vi "02reg_path_file.vi"(1 "Nombre":string, 2 "Nº equipo":i32, 3 "Exe path":string) -> (0 "file path nvo":path=path "C:/Documents and Settings/All Users/Documentos/LabVIEW Data/Soft Telemedicion/Beta 2.2/Equipo1/09-06-18.xls")   [LabVIEW 2010]
uses:
  <vilib>/Utility/file.llb/Read From Spreadsheet File (DBL).vi
panel:
  out "error out":errorcluster
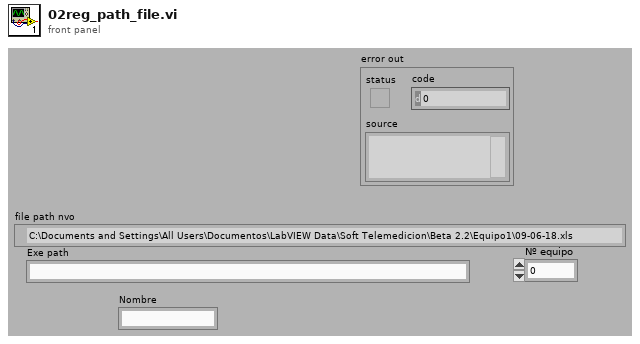
[diagram p1: front panel]
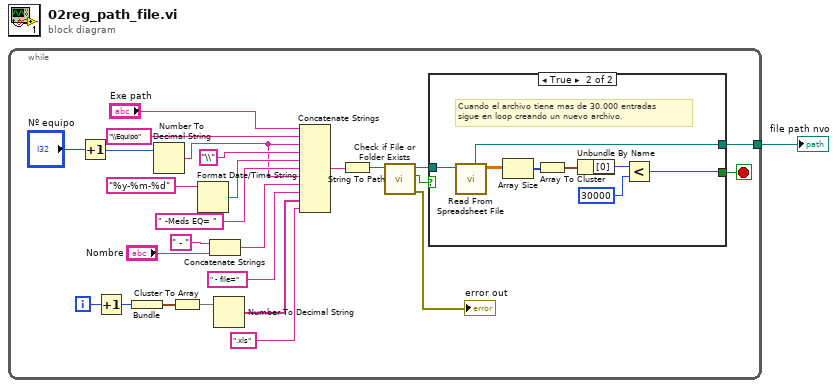
[diagram p0: block diagram]
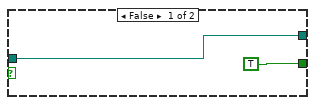
[diagram p2: hidden frame]
diagram:
  n1 = while {
    tunnel: [w18] -> w1
    i -> [w20]
    stop <- w19 stop-if-true
    n2 = Increment(x="Nº equipo") -> (x+1=w10:i32)
    n3 = Increment(x=w20) -> (x+1=w16:i32)
    n4 = Bundle(w16) -> (w24:cluster{i32})  [unwired: 1 in]
    n5 = Number To Decimal String(number=w10) -> (decimal integer string=w9:string)  [unwired: 1 out]
    n6 = Cluster To Array(cluster=w24) -> (array=w17:i32[])
    n7 = Format Date/Time String(time format string (%c)="%y-%m-%d") -> (date/time string=w26:string)  [unwired: 2 out]
    n8 = Concatenate Strings(" - " ("time format string (%c)"), "Nombre") -> (w7:string)
    n9 = Number To Decimal String(number=w17) -> (decimal integer string=w5:string[])  [unwired: 1 out]
    n10 = Concatenate Strings("Exe path", "\\Equipo" ("replace string (\"\")"), w9, "\\" ("time format string (%c)"), w26, " -Meds EQ= " ("string"), w9, w7, " - file=" ("string"), w5, ".xls" ("string")) -> (w12:string)
    n11 = String To Path(string=w12) -> (path=w23:path)
    n12 = call <vilib>:"Check if File or Folder Exists.vi"("path"=w23) -> ("error out"=→"error out":errorcluster, "file or folder exists?"=w22:bool, "dup path"=w21:path)  [unwired: 1 in, 7 out]
    n13 = case shown="True" w22 {
      tunnel: w21 -> [w28 w32]
      tunnel: [TRUE w31] -> w19
      tunnel: [w28 w30] -> w18
      frame False {
      }
      frame True {
        # "Cuando el archivo tiene mas de 30.000 entradas\nsigue en loop creando un nuevo archivo."
        n14 = call-poly <vilib>:"Read From Spreadsheet File.vi"("file path (dialog if empty)"=w32) -> ("all rows"=w35:dbl[][], "new file path (Not A Path if cancelled)"=w30:path)  [unwired: 3 in, 6 out]
        n15 = Array Size(array=w35) -> (size(s)=w34:i32[])
        n16 = Array To Cluster(array=w34) -> (cluster=w33:cluster{"[0]":i32})
        n17 = Unbundle By Name(w33) -> ("[0]"=w36:i32)
        n18 = Less?(x=w36, y=30000) -> (x < y?=w31:bool)
      }
    }
  }
  "file path nvo" <- w1
